vi "AlazarOCTIgnoreBadClock.vi"(0 "Handle":u32, 5 "Enable":u32, 7 "Good Clock Duration":dbl, 9 "Bad Clock Duration":dbl, 11 "error in (no error)":errorcluster) -> (4 "Handle":u32, 6 "Trigger Cycle Time":dbl, 8 "Trigger Pulse Width":dbl, 10 "Return Code":u32, 15 "error out":errorcluster)   [LabVIEW 2021]
doc: "Get a board model identifier of the board associated with a board handle."
uses:
  ATSApi.dll
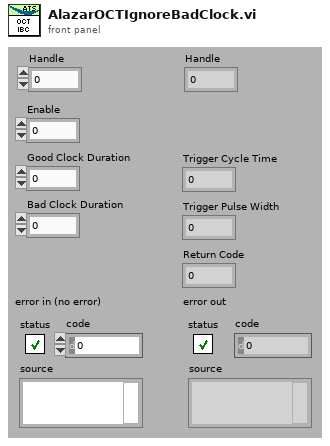
[diagram p1: front panel]
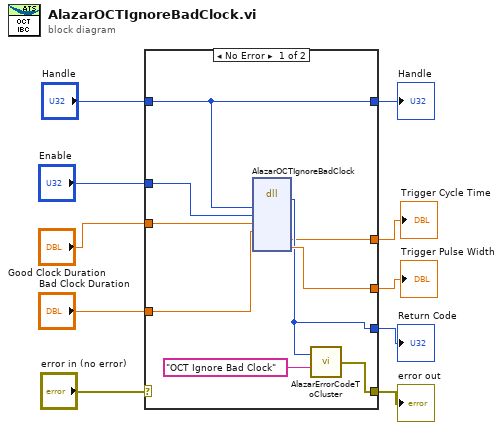
[diagram p0: block diagram]
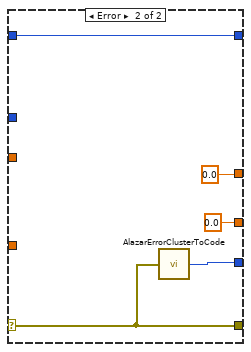
[diagram p2: hidden frame]
diagram:
  n1 = case shown="No Error" "error in (no error)" {
    selector: "error in (no error)" -> [_ w24]
    tunnel: [w13 w24] -> w9
    tunnel: [w12 w23] -> w8
    tunnel: "Handle" -> [w19 w22]
    tunnel: [w19 w22] -> w6
    tunnel: "Enable" -> [w18 _]
    tunnel: "Good Clock Duration" -> [w17 _]
    tunnel: "Bad Clock Duration" -> [w16 _]
    tunnel: [w15 0.0] -> w2
    tunnel: [w11 0.0] -> w1
    frame No Error {
      n2 = dll-call lib="ATSApi.dll" fn="AlazarOCTIgnoreBadClock"("handle"=w19, "enable"=w18, "goodClockDuration"=w17, "badClockDuration"=w16) -> (w12:u32, "triggerCycleTime"=w11:dbl, "triggerPulseWidth"=w15:dbl)  [unwired: 9 in, 2 out]
      n3 = call "AlazarErrorCodeToCluster.vi"("Message"="OCT Ignore Bad Clock", "Error Code"=w12) -> ("error out"=w13:errorcluster)
    }
    frame Error {
      n4 = call "AlazarErrorClusterToCode.vi"("error in (no error)"=w24) -> ("Error Code"=w23:u32)
    }
  }
  "Handle" <- w6
  "error out" <- w9
  "Return Code" <- w8
  "Trigger Cycle Time" <- w1
  "Trigger Pulse Width" <- w2
